vi "Set Dev Notice Event.vi"(10 "rmvevent":u32, 11 "addevent":u32) -> (2 "rmvevent out":u32, 3 "addevent out":u32)   [LabVIEW 2021, in "vmmso.lvlib"]
doc: "DLL_API void WINAPI SetDevNoticeEvent(HANDLE addevent, HANDLE rmvevent);"
uses:
  vmmso.lvlib
  vmmso.dll
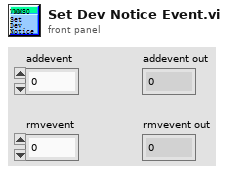
[diagram p1: front panel]
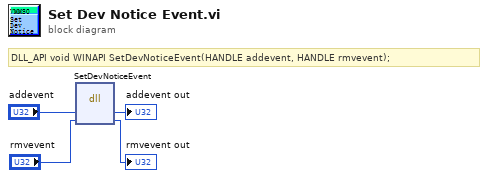
[diagram p0: block diagram]
diagram:
  # "DLL_API void WINAPI SetDevNoticeEvent(HANDLE addevent, HANDLE rmvevent);"
  n1 = dll-call lib="D:/labviewdemo/LabviewDemo 21/vmmso/vmmso.*" fn="SetDevNoticeEvent"("addevent"="addevent", "rmvevent"="rmvevent") -> ("addevent"=→"addevent out":u32, "rmvevent"=→"rmvevent out":u32)  [unwired: 4 in, 2 out]
